vi "CMD_GETVAC.vi"(6 "Gantry in":refnum<class "Gantry.lvclass">, 8 "error in (no error)":errorcluster, 10 "Arguments":string[](array[string]), 11 "gScript Interpreter in":refnum<class "gScript Interpreter.lvclass">) -> (0 "error out":errorcluster, 3 "gScript Interpreter out":refnum<class "gScript Interpreter.lvclass">, 4 "Gantry out":refnum<class "Gantry.lvclass">)   [LabVIEW 2024, in "gScript Interpreter.lvclass"]
uses:
  gScript Interpreter.lvclass
  Shared Components/Gantry Class/Gantry.lvclass
  Type Definitions/Memory Cell.ctl
  Type Definitions/Memory Cell Type Enum.ctl
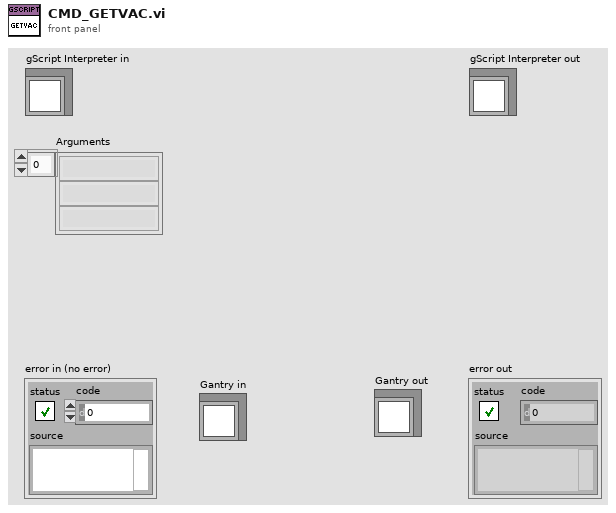
[diagram p1: front panel]
types:
  T1 = typedef "Memory Cell Type Enum.ctl" = enum16{"integer", "float", "vector", "rotation"}
  T2 = typedef "Memory Cell.ctl" = cluster{"type":T1, "x":dbl, "y":dbl, "z":dbl, "w":dbl}
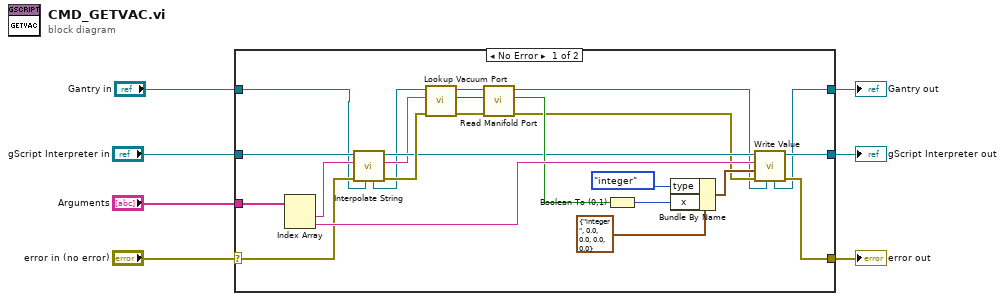
[diagram p0: block diagram]
diagram:
  n1 = case shown="No Error" "error in (no error)" {
    selector: "error in (no error)" -> [w17 w33]
    tunnel: [w12 w33] -> w6
    tunnel: [w25 w32] -> w4
    tunnel: "gScript Interpreter in" -> [w19 w32]
    tunnel: "Arguments" -> [w30 _]
    tunnel: "Gantry in" -> [w9 w31]
    tunnel: [w10 w31] -> w1
    frame No Error {
      n2 = Index Array(array=w30) -> (element #1=w18:string, element #2=w29:string)  [unwired: 2 in]
      n3 = call-dynamic "Interpolate String.vi"("Gantry in"=w9, "error in (no error)"=w17, "Input String"=w18, "gScript Interpreter in"=w19) -> ("error out"=w16:errorcluster, "Output String"=w14:string, "gScript Interpreter out"=w15:refnum<class "gScript Interpreter.lvclass">, "Gantry out"=w8:refnum<class "Gantry.lvclass">)  [unwired: 4 in]
      n4 = call-dynamic "Lookup Vacuum Port.vi"("error in (no error)"=w16, "Channel Name"=w14, "Gantry Class in"=w8) -> ("error out"=w27:errorcluster, "Port Number"=w26:i32, "Gantry Class out"=w28:refnum<class "Gantry.lvclass">)  [unwired: 5 in]
      n5 = call-dynamic "Read Manifold Port.vi"("error in"=w27, "Manifold Port"=w26, "Gantry in"=w28) -> ("error out"=w13:errorcluster, "On/Off"=w22:bool, "Gantry out"=w11:refnum<class "Gantry.lvclass">)  [unwired: 6 in]
      n6 = Boolean To (0,1)(Boolean=w22) -> (0, 1=w21:i16)
      n7 = Bundle By Name(cluster=T2 {"type"=enum."integer", "x"=0.0, "y"=0.0, "z"=0.0, "w"=0.0} ("Value"), "type"=Memory_Cell_Type_Enum."integer", "x"=w21) -> (w23:T2)
      n8 = call-dynamic "Write Value.vi"("Gantry in"=w11, "error in (no error)"=w13, "Value"=w23, "Address"=w29, "gScript Interpreter in"=w15) -> ("error out"=w12:errorcluster, "gScript Interpreter out"=w25:refnum<class "gScript Interpreter.lvclass">, "Gantry out"=w10:refnum<class "Gantry.lvclass">)  [unwired: 4 in]
    }
    frame Error {
    }
  }
  "error out" <- w6
  "gScript Interpreter out" <- w4
  "Gantry out" <- w1
